vi "Read Pin.vi"(0 "NXP in":refnum<class "NXP.lvclass">, 5 "VISA resource name":refnum<visa-resource-name>, 9 "Port":dbl, 11 "error in (no error)":errorcluster) -> (4 "NXP out":refnum<class "NXP.lvclass">, 6 "VISA resource name 2":refnum<visa-resource-name>, 8 "Pin":bool, 10 "Response":string, 15 "error out":errorcluster)   [LabVIEW 2020, in "NXP.lvclass"]
uses:
  NXP.lvclass
  f13a5b9d-1546-4342-a960-20c63ba04679.vi
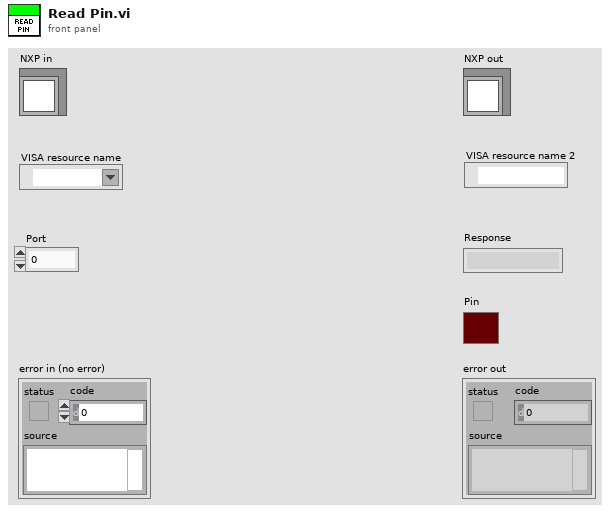
[diagram p1: front panel]
types:
  T1 = enum16{"Write", "Read", "Config", "Reset", "Close"}
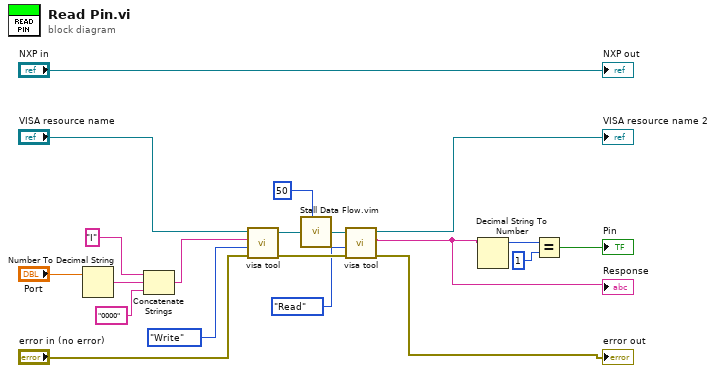
[diagram p0: block diagram]
diagram:
  n1 = Number To Decimal String(number="Port") -> (decimal integer string=w16:string)  [unwired: 1 in]
  n2 = Concatenate Strings("I" ("string"), w16, "0000" ("string")) -> (w15:string)
  n3 = call "visa tool.vi"("error in (no error)"="error in (no error)", "Opciones"=T1."Write", "Write"=w15, "VISA com port"="VISA resource name") -> ("error out"=w13:errorcluster, "VISA com port 2"=w3:refnum<visa-resource-name>)  [unwired: 5 in, 1 out]
  n4 = call "Stall Data Flow.vim"("value in"=w3, "milliseconds to wait"=u32 50) -> ("value out"=w2:refnum<visa-resource-name>)  [unwired: 1 out]
  n5 = call "visa tool.vi"("error in (no error)"=w13, "Opciones"=T1."Read", "VISA com port"=w2) -> ("error out"=→"error out":errorcluster, "Read"=w8:string, "VISA com port 2"=→"VISA resource name 2":refnum<visa-resource-name>)  [unwired: 6 in]
  "Response" <- w8
  n6 = Decimal String To Number(string=w8) -> (offset past number=w18:i32)  [unwired: 2 in, 1 out]
  n7 = Equal?(x=w18, y=1) -> (x = y?=→"Pin":bool)
  "NXP out" <- "NXP in"
